vi "Game_SolvePuzzle.vi"(8 "error in (no error)":errorcluster, 10 "Guess":string, 11 "Solution":string) -> (0 "error out":errorcluster, 2 "Correct":bool, 3 "Solution OUT":string)   [LabVIEW 2020]
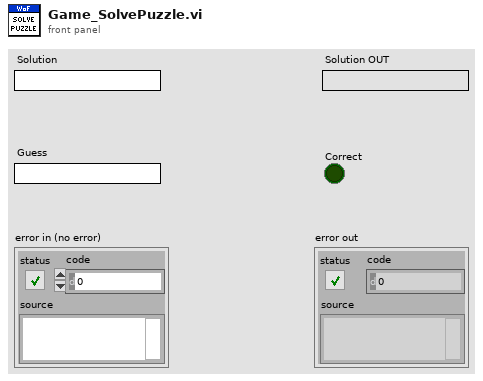
[diagram p1: front panel]
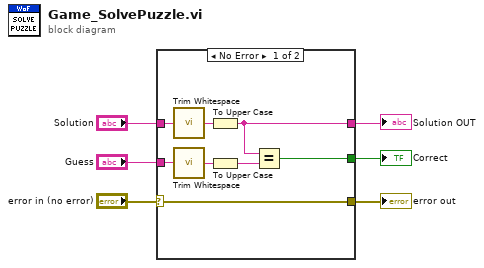
[diagram p0: block diagram]
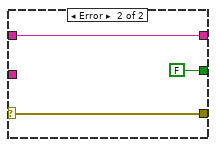
[diagram p2: hidden frame]
diagram:
  n1 = case shown="No Error" "error in (no error)" {
    selector: "error in (no error)" -> [w8 w15]
    tunnel: "Guess" -> [w13 _]
    tunnel: "Solution" -> [w14 w17]
    tunnel: [w9 w17] -> w3
    tunnel: [w8 w15] -> w2
    tunnel: [w7 FALSE] -> w1
    frame No Error {
      n2 = call <vilib>:"Trim Whitespace.vi"("string"=w14) -> ("trimmed string"=w12:string)  [unwired: 1 in]
      n3 = call <vilib>:"Trim Whitespace.vi"("string"=w13) -> ("trimmed string"=w11:string)  [unwired: 1 in]
      n4 = To Upper Case(1:w12) -> (0:w9:string)
      n5 = To Upper Case(1:w11) -> (0:w10:string)
      n6 = Equal?(x=w9, y=w10) -> (x = y?=w7:bool)
    }
    frame Error {
    }
  }
  "error out" <- w2
  "Solution OUT" <- w3
  "Correct" <- w1
